vi "Read Macros List.vi"(11 "Motions in":refnum<class "Motions.lvclass">) -> (2 "Macros List":cluster{"enabled?":bool, "macro name":string}[](array[cluster]), 3 "Motions out":refnum<class "Motions.lvclass">)   [LabVIEW 2016, in "Hardware.lvlib" / "Motions.lvlib" / "Motions.lvclass"]
uses:
  <userlib>/Common Components/Hardware/Abstract System/Motions/Motions/Motions.lvclass
  <userlib>/Common Components/Hardware/Abstract System/Motions/Motions/Motions.lvclass/Motions.ctl
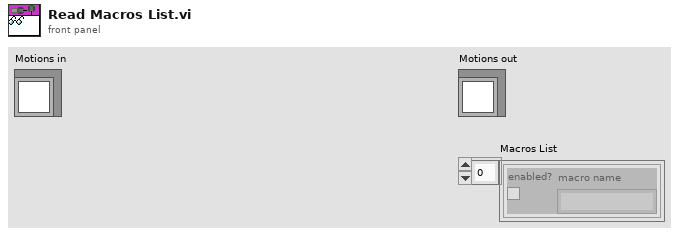
[diagram p1: front panel]
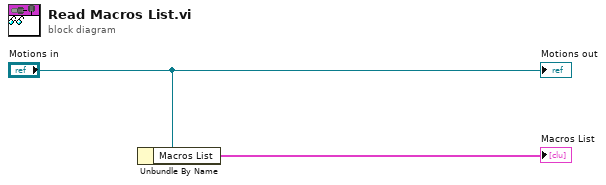
[diagram p0: block diagram]
diagram:
  n1 = Unbundle By Name("Motions in") -> ("Macros List"=→"Macros List":cluster{"enabled?":bool, "macro name":string}[])
  "Motions out" <- "Motions in"
